vi "TTTRHDR_H_write.vi"(8 "error in (no error)":errorcluster, 10 "TTTRHDR_H":T1, 11 "refnum in":refnum<file>) -> (0 "error out":errorcluster, 3 "refnum out":refnum<file>)   [LabVIEW 2012]
uses:
  TTTR_data_headers/TTTRHDR_H.ctl
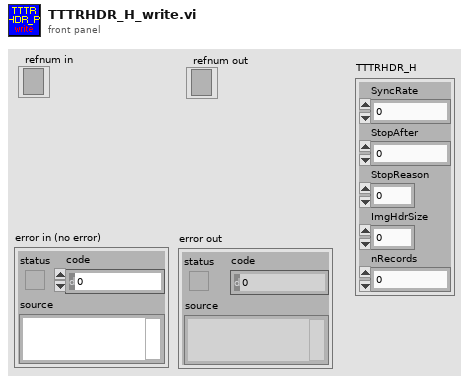
[diagram p1: front panel]
types:
  T1 = typedef "TTTRHDR_H.ctl" = cluster{"SyncRate":i32, "StopAfter":i32, "StopReason":i32, "ImgHdrSize":i32, "nRecords":u64}
  T2 = enum16{"big-endian, network order", "native, host order", "little-endian"}
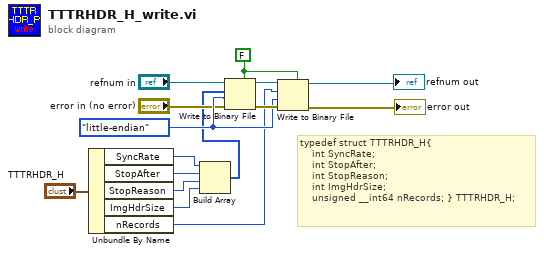
[diagram p0: block diagram]
diagram:
  w7 = FALSE ("prepend array or string size? (T)")
  w13 = T2."little-endian" ("byte order (0:big-endian, network order)")
  # "typedef struct TTTRHDR_H{\t\n\t\t\t\tint SyncRate;\n\t\t\t\tint StopAfter;\n\t\t\t\tint StopReason;\n\t\t\t\tint ImgHdrSize;\n\t\t\t\tunsigned __int64 nRecords;\t} TTTRHDR_H;"
  n1 = Unbundle By Name("TTTRHDR_H") -> ("SyncRate"=w6:i32, "StopAfter"=w5:i32, "StopReason"=w4:i32, "ImgHdrSize"=w3:i32, "nRecords"=w2:u64)
  n2 = Build Array(w6, w5, w4, w3) -> (w1:i32[])
  n3 = Write to Binary File(file (use dialog)="refnum in", data=w1, error in="error in (no error)", 5:w7, 9:w13) -> (refnum out=w14:refnum<file>, error out=w15:errorcluster)  [unwired: 1 in, 1 out]
  n4 = Write to Binary File(file (use dialog)=w14, data=w2, error in=w15, 5:w7, 9:w13) -> (refnum out=→"refnum out":refnum<file>, error out=→"error out":errorcluster)  [unwired: 1 in, 1 out]
